vi "Reset Resource.vi"(6 "Remote Timeout (300,000 ms)":u32=300000, 8 "error in (no error)":errorcluster, 10 "Reset Mode (hardware)":u32(ring) items=["reinitialize hardware", "clear software settings"], 11 "Resource in":refnum<k20>) -> (0 "error out":errorcluster, 2 "Detailed Result":string, 3 "Resource out":refnum<k20>, 4 "Dependent Items Deleted":bool)   [LabVIEW 2020, in "nisyscfg.lvlib"]
doc: "Executes reset on a specified resource. By default, it reinitializes the hardware to its power-on state."
uses:
  <vilib>/nisyscfg/nisyscfg.lvlib
  <vilib>/Utility/error.llb/Error Cluster From Error Code.vi
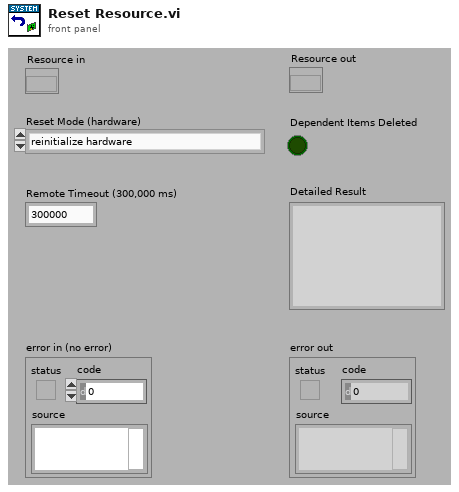
[diagram p1: front panel]
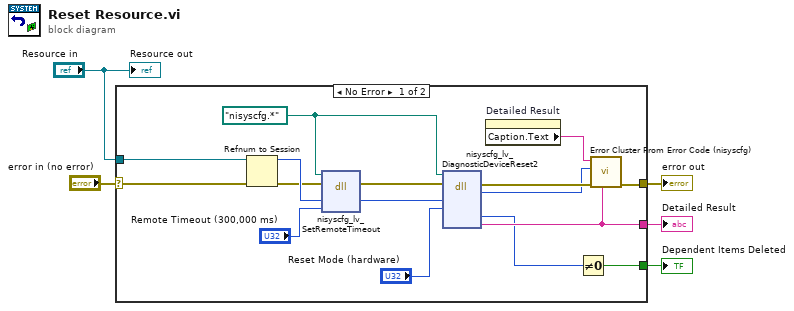
[diagram p0: block diagram]
diagram:
  n1 = case shown="No Error" "error in (no error)" {
    selector: "error in (no error)" -> [w15 w22]
    tunnel: [w11 w22] -> w5
    tunnel: "Resource in" -> [w14 _]
    tunnel: [w9 _] -> w2
    tunnel: [w8 _] -> w1
    frame No Error {
      w13 = path "nisyscfg.*" ("path in")
      n2 = Refnum to Session(4:w15, 7:w14) -> (0:w16:errorcluster, 3:w18:u64)
      n3 = dll-call lib="nisyscfg.*" fn="nisyscfg_lv_SetRemoteTimeout" label="SetRemoteTimeout"(path in=w13, error in=w16, "item"=w18, "connectTimeout"="Remote Timeout (300,000 ms)") -> (error out=w19:errorcluster, "item"=w17:u64)  [unwired: 1 in, 3 out]
      n4 = dll-call lib="nisyscfg.*" fn="nisyscfg_lv_DiagnosticDeviceReset2" label="DiagnosticDeviceReset2"(path in=w13, error in=w19, "item"=w17, "mode"="Reset Mode (hardware)") -> (error out=w12:errorcluster, "status"=w10:i32, "moreDeleted"=w7:u8, "detailedResult"=w9:string)  [unwired: 4 in, 2 out]
      n5 = property on="Detailed Result" class="Str"() -> ("Caption.Text"=w6:string)  [unwired: 2 in, 2 out]
      n6 = Not Equal To 0?(x=w7) -> (x != 0?=w8:bool)
      n7 = call <vilib>:"Error Cluster From Error Code (nisyscfg).vi"("Details String"=w9, "error in (no error)"=w12, "Error Code (0)"=w10, "Details Caption"=w6) -> ("error out"=w11:errorcluster)  [unwired: 7 in]
    }
    frame Error {
    }
  }
  "error out" <- w5
  "Detailed Result" <- w2
  "Dependent Items Deleted" <- w1
  "Resource out" <- "Resource in"
